vi "Patient info Dialog.vi"() -> (2 "OK":bool)   [LabVIEW 2015]
panel:
  in  "Cancel Button":bool
  in  "OK Button":bool
  in  "EyeColor 2":u16(ring) caption="Treated Eye:" items=["Right", "Left"]
  in  "EyeColor":u16(ring) caption="Eye Color:" items=["Brown", "Green", "Blue", "Black"]
  in  "PatientGender":enum32{"Male", "Female"}(radio) caption="Gender:"
  in  "PatientAge":dbl caption="Age:"
  in  "PatientName":string caption="Name:"
  # "Patient Information Editor"
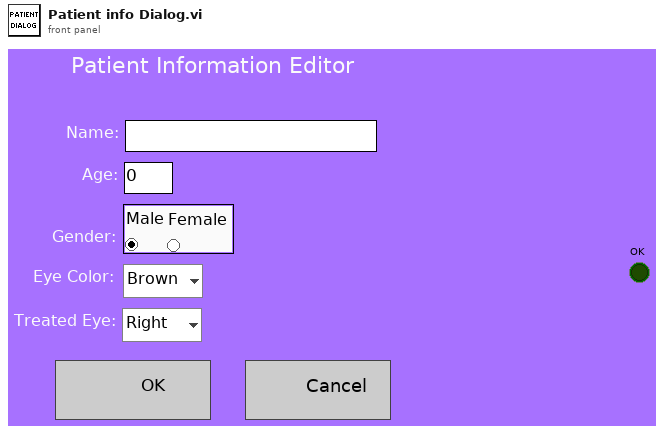
[diagram p1: front panel]
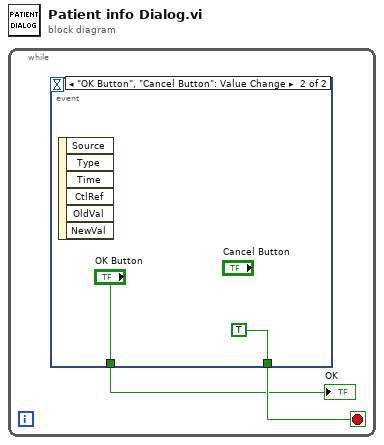
[diagram p0: block diagram]
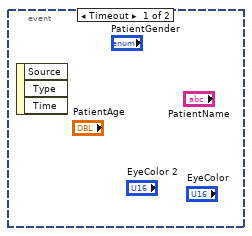
[diagram p2: hidden frame]
diagram:
  n1 = while {
    stop <- w2 stop-if-true
    n2 = event shown="[1] \"OK Button\", \"Cancel Button\": Value Change" {
      selector: _ -> [_ _]
      dyn-events: _ -> [_ _]
      timeout: _ -> [_ _]
      tunnel: [_ TRUE] -> w2
      tunnel: [_ "OK Button"] -> w1
      event Timeout {
        n3 = event-data() -> ()  [unwired: 1 in, 3 out]
      }
      event "OK Button", "Cancel Button": Value Change {
        n4 = event-data() -> ()  [unwired: 1 in, 6 out]
      }
    }
    "OK" <- w1
  }
